vi "scaler64_analog.vi"(0 "Enable_SCALER":bool, 2 "OneShot_SCALER":bool, 3 "SampleAnalog_SCALER":bool, 5 "Gate_SCALER":bool[](array[boolean])=[FALSE, FALSE, FALSE, FALSE, FALSE], 8 "PresetValues_SCALER":u32[](array[numeric])=[0, 0, 0, 0, 0], 9 "AnalogInputs_SCALER":fxp<+/-,20,5>[](array[numeric])=[0.0, 0.0, 0.0, 0.0], 10 "fxp_ShiftLeft_SCALER":u64, 11 "divisor_SCALER":u32=4) -> (13 "fxp_ScaledAI_SCALER":u64[](array[numeric]), 14 "Done_SCALER":bool, 15 "fxp_RawAI0_SCALER":u64, 16 "fxp_RawAI1_SCALER":u64, 17 "fxp_RawAI2_SCALER":u64, 18 "fxp_RawAI3_SCALER":u64, 19 "Counter_SCALER":u32[](array[numeric]))   [LabVIEW 2019, in "scaler.lvlib"]
uses:
  scaler.lvlib
  Cast-EPICS/cast u64 to s-64-64.vi
  Cast-EPICS/cast s-64-32 to u64.vi
  Cast-EPICS/fixedpoint-cast.lvlib
panel:
  # "This is a 64 channel analog scaler. It follows to the word the definition of the scaler in the anl website\nhttps://epics.anl.gov/bcda/synApps/std/scalerRecord.html"
  # "Input and output description\n - Gate_Scaler[64] : corresponds to 64 counters S1-S64\n - SampleAnalog_Scaler[63] : corresponds to 63 counters S2-S64\n - PresetValues_Scaler[64]: corresponds to 64 counters S1-S64\n - OneShot_Scaler: Oneshot / autocount is also implemented \n                                 in hardware. When necessary, can be used.\n                                 When not necessary (implmented in software)\n                                 this port can be fixed to 1.\n - AnalogInputs_Scaler[63] : The inputs to be summed when the\n                                                 corresponding Pulse_Scaler transits \n                                                 from 0 -> 1. (S2-S64)\n - Counter_Scaler[64]: 64 counter readings.\n - Done_Scaler : Done signal as per Scaler specifications\n - Enable_Scaler: Set to one when CNT is set to 1.\n-  Divisor_Scaler: If not set to 1, the S1 counter will increment every\n                             \"Divisor\" ticks.\n- ao_ShiftLeft_SCALER : This parameter shifts all the voltage readings\n                                          by a value. Postive is shift left, and negative is\n                                          shift right."
  # "Optimization tip:\nMake all the arrays the same size as the number\nof channels you need implemented. Setting\nthe number of channels uses up to 45% of the \nresources. Setting to 2 uses only 23%."
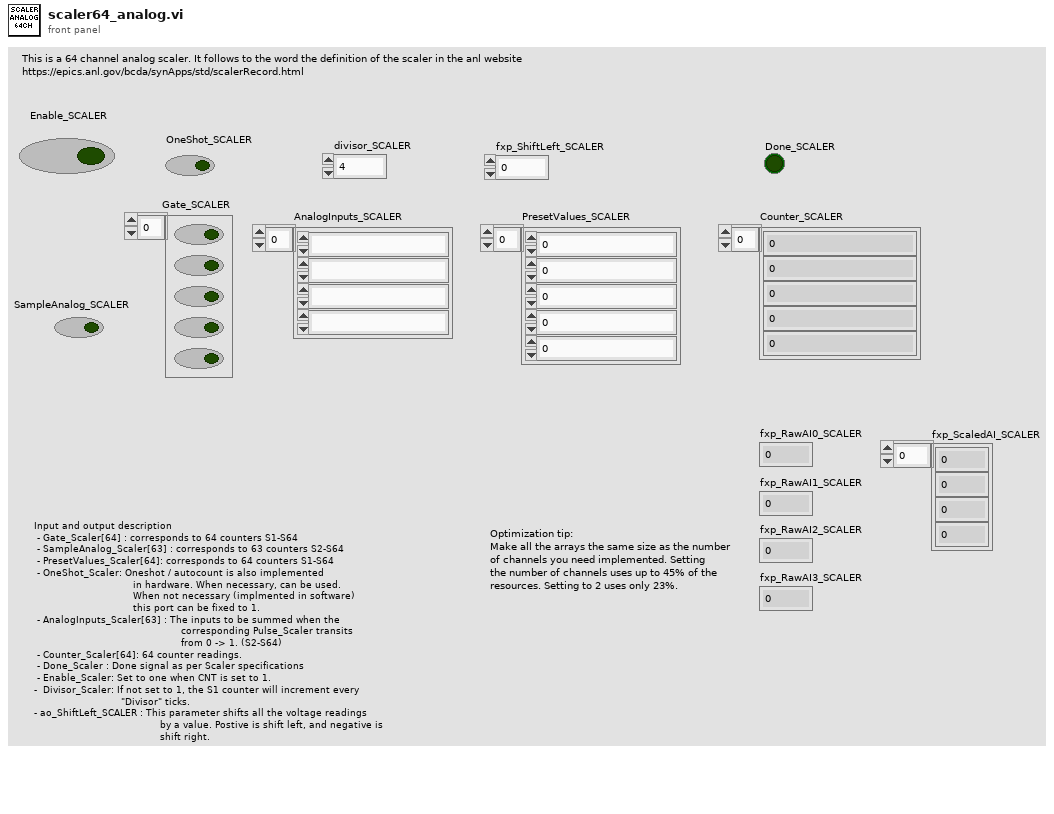
[diagram p1: front panel]
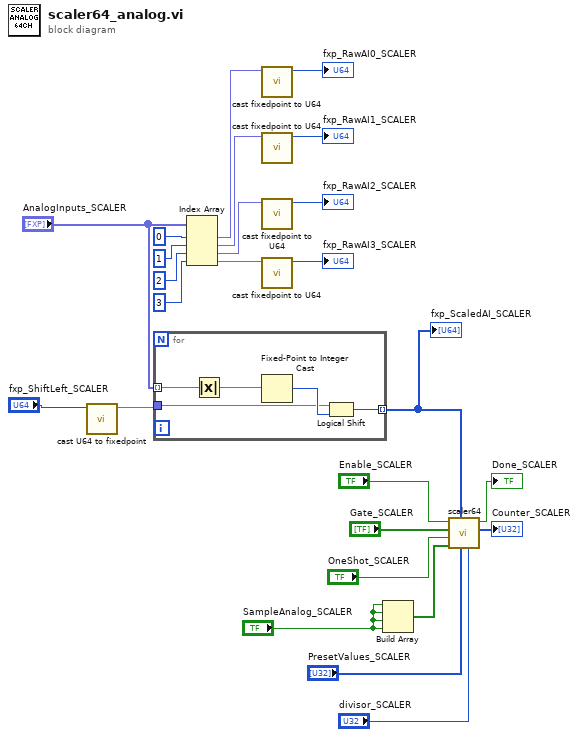
[diagram p0: block diagram]
diagram:
  n1 = call-poly "cast U64 to fixedpoint.vi"("aofxp"="fxp_ShiftLeft_SCALER") -> ("fixedpoint_o"=w2:fxp<+/-,64,64>)  [unwired: 10 in]
  n2 = for {
    tunnel: "AnalogInputs_SCALER" -> [w29] mode=indexing
    tunnel: [w27] -> w1 mode=indexing
    tunnel: w2 -> [w26]
    n3 = Absolute Value(x=w29) -> (abs(x)=w30:fxp<+,20,5>)
    n4 = Fixed-Point to Integer Cast(1:w30) -> (0:w28:u32)
    n5 = Logical Shift(y=w26, x=w28) -> (x << y=w27:u32)
  }
  "fxp_ScaledAI_SCALER" <- w1
  n6 = Index Array(array="AnalogInputs_SCALER", index #1=i16 0, index #2=i16 1, index #3=i16 2, index #4=i16 3) -> (element #1=w11:fxp<+/-,20,5>, element #2=w9:fxp<+/-,20,5>, element #3=w8:fxp<+/-,20,5>, element #4=w7:fxp<+/-,20,5>)
  n7 = call-poly "cast fixedpoint to U64.vi"("fixedpoint_i"=w11) -> ("aifxp"=→"fxp_RawAI0_SCALER":u64)  [unwired: 10 in]
  n8 = call-poly "cast fixedpoint to U64.vi"("fixedpoint_i"=w9) -> ("aifxp"=→"fxp_RawAI1_SCALER":u64)  [unwired: 10 in]
  n9 = call-poly "cast fixedpoint to U64.vi"("fixedpoint_i"=w8) -> ("aifxp"=→"fxp_RawAI2_SCALER":u64)  [unwired: 10 in]
  n10 = call-poly "cast fixedpoint to U64.vi"("fixedpoint_i"=w7) -> ("aifxp"=→"fxp_RawAI3_SCALER":u64)  [unwired: 10 in]
  n11 = Build Array("SampleAnalog_SCALER", "SampleAnalog_SCALER", "SampleAnalog_SCALER", "SampleAnalog_SCALER") -> (w13:bool[])
  n12 = call "scaler64.vi"("divisor_Scaler"="divisor_SCALER", "PresetValues_Scaler"="PresetValues_SCALER", "AnalogInputs_Scaler"=w1, "Pulse_Scaler"=w13, "OneShot_Scaler"="OneShot_SCALER", "Gate_Scaler"="Gate_SCALER", "Enable_Scaler"="Enable_SCALER") -> ("Counter_Scaler"=→"Counter_SCALER":u32[], "Done_Scaler"=→"Done_SCALER":bool)  [unwired: 3 in]
